vi "Shooter Speed Global.vi"() -> ()   [LabVIEW 2011]
panel:
  out "Hood Voltage":dbl
  out "Indexer Set Speed":dbl
  out "ShooterSet Speed":dbl
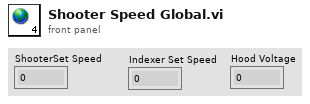
[diagram p1: front panel]
diagram:
